vi "ReceivePacket.vi"(6 "error in":errorcluster, 9 "connection ID":refnum<k5>) -> (0 "error out":errorcluster, 3 "connection ID out":refnum<k5>, 4 "payload":string)   [LabVIEW 2014, in "Raspberry Pi Compatible Compiler for LabVIEW.lvlib" / "Websocket.lvlib"]
uses:
  Websocket.lvlib
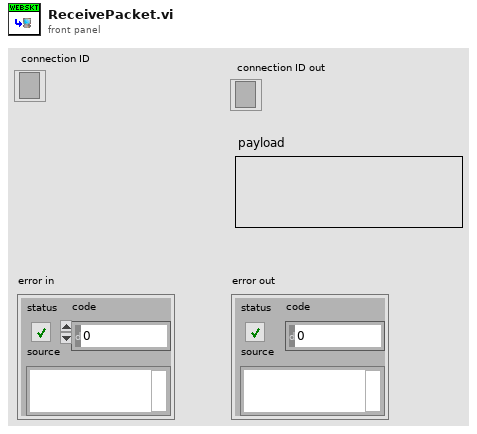
[diagram p1: front panel]
types:
  T1 = typedef "Raspberry Pi Compatible Compiler for LabVIEW.lvlib/Websocket.lvlib/WebsocketFrameTypes_TD.ctl" = enum8{"Continuation", "Text", "Binary", "Reserved 1", "Reserved 2", "Reserved 3", "Reserved 4", "Reserved 5", "Close", "Ping", "Pong", "Reserved 6", "Reserved 7", "Reserved 8", "Reserved 9", "Reserved 10"}
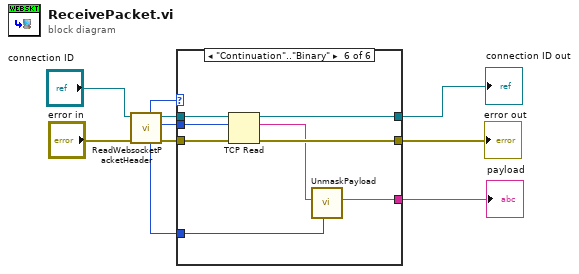
[diagram p0: block diagram]
diagram:
  n1 = call "ReadWebsocketPacketHeader.vi"("error in"="error in", "connection ID"="connection ID") -> ("error out"=w8:errorcluster, "payload length"=w9:u64, "connection ID out"=w7:refnum<k5>, "mask value"=w2:u32, "opcode"=w10:T1)  [unwired: 3 in, 2 out]
  n2 = case shown="\"Continuation\"..\"Binary\"" w10 {
    tunnel: w7 -> [w12 w13 w16 w18 w20 w28]
    tunnel: w8 -> [w11 w14 w15 w17 w19 w27]
    tunnel: w9 -> [_ _ _ _ _ w26]
    tunnel: [w12 w13 w16 w18 w20 w25] -> w5
    tunnel: [w11 w14 w15 w17 w19 w24] -> w6
    tunnel: w2 -> [_ _ _ _ _ w21]
    tunnel: [_ _ _ _ _ w22] -> w1
    frame "Reserved 1".."Reserved 5" {
    }
    frame "Close" {
    }
    frame "Ping" {
    }
    frame "Pong" {
    }
    frame "Reserved 6".."Reserved 10" {
    }
    frame "Continuation".."Binary" {
      n3 = TCP Read(connection ID=w28, bytes to read=w26, error in (no error)=w27) -> (connection ID out=w25:refnum<k5>, data out=w23:string, error out=w24:errorcluster)  [unwired: 2 in]
      n4 = call "UnmaskPayload.vi"("mask value"=w21, "payload"=w23) -> ("unmasked payload"=w22:string)  [unwired: 7 in]
    }
  }
  "connection ID out" <- w5
  "error out" <- w6
  "payload" <- w1
